vi "Is Resource Available.vi"(9 "Data":string, 11 "WebSocket Connection in":refnum<class "WebSocket Connection.lvclass">) -> (0 "Is Service Available":bool, 1 "Data Out":string, 3 "WebSocket Connection out":refnum<class "WebSocket Connection.lvclass">)   [LabVIEW 2016, in "WebSocket Actors.lvlib" / "WebSocket Connection.lvclass"]
uses:
  WebSocket Connection.lvclass
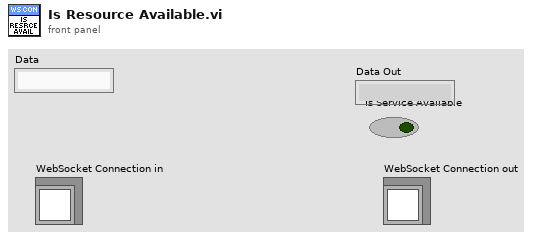
[diagram p1: front panel]
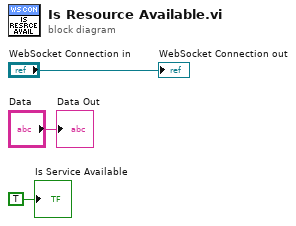
[diagram p0: block diagram]
diagram:
  "Is Service Available" <- TRUE ("Is Service Available")
  "Data Out" <- "Data"
  "WebSocket Connection out" <- "WebSocket Connection in"
